vi "Delete Header from NoteID.vi"(7 "Actor Name":string, 11 "node ID full name":string) -> (3 "node ID delete header ns=2;s=":string)   [LabVIEW 2021]
doc: "ns=2;s=Model_UI.ModelName\nfull name NoteID come in , the header \"ns=2;3=\", will be delete."
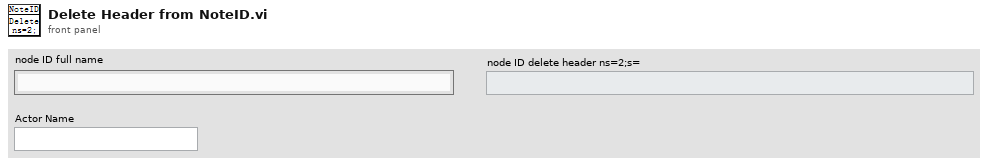
[diagram p1: front panel]
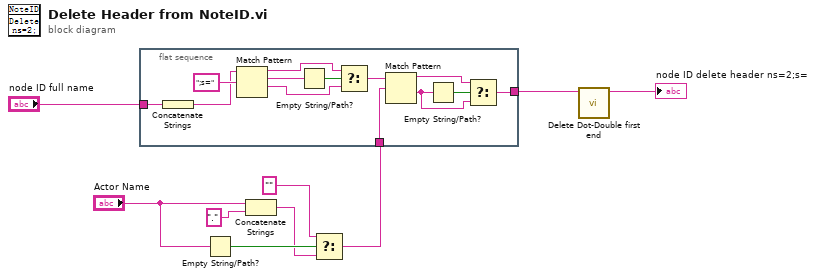
[diagram p0: block diagram]
diagram:
  n1 = flat-sequence {
    tunnel: [w12] -> w7
    tunnel: "node ID full name" -> [w11]
    tunnel: w2 -> [w10]
    frame #0 {
      n2 = Concatenate Strings(w11) -> (w13:string)
      n3 = Match Pattern(string=w13, regular expression=";s=") -> (before substring=w16:string, match substring=w18:string, after substring=w15:string)  [unwired: 1 in, 1 out]
      n4 = Empty String/Path?(string/path=w18) -> (empty?=w17:bool)
      n5 = Select(t=w16, s=w17, f=w15) -> (s? t:f=w14:string)
      n6 = Match Pattern(string=w14, regular expression=w10) -> (before substring=w21:string, after substring=w22:string)  [unwired: 1 in, 2 out]
      n7 = Empty String/Path?(string/path=w22) -> (empty?=w20:bool)
      n8 = Select(t=w21, s=w20, f=w22) -> (s? t:f=w12:string)
    }
  }
  n9 = Empty String/Path?(string/path="Actor Name") -> (empty?=w5:bool)
  n10 = Concatenate Strings("Actor Name", "." ("regular expression")) -> (w3:string)
  n11 = Select(t="", s=w5, f=w3) -> (s? t:f=w2:string)
  n12 = call "Delete Dot-Double first end.vi"("String"=w7) -> ("string"=→"node ID delete header ns=2;s=":string)  [unwired: 10 in]
